vi "GetFrameRate.vi"(8 "error in (no error)":errorcluster, 11 "ICamera in":refnum<class "ICamera.lvclass">) -> (0 "error out":errorcluster, 2 "Frame Rate":u8 format="%.0x", 3 "ICamera out":refnum<class "ICamera.lvclass">)   [LabVIEW 2020, in "ICamera.lvlib" / "ICamera.lvclass"]
uses:
  ICamera.lvclass
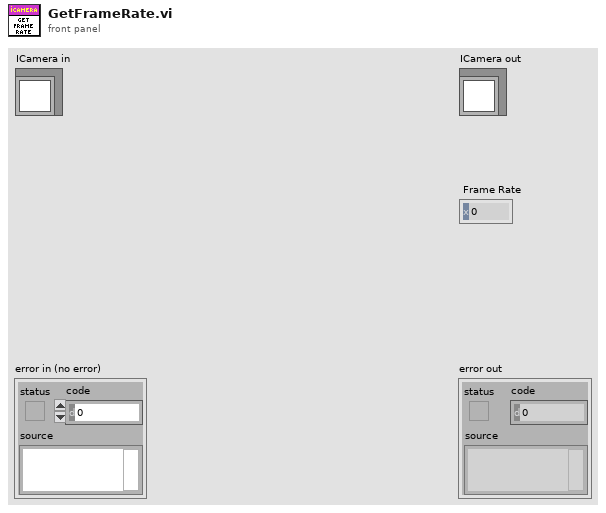
[diagram p1: front panel]
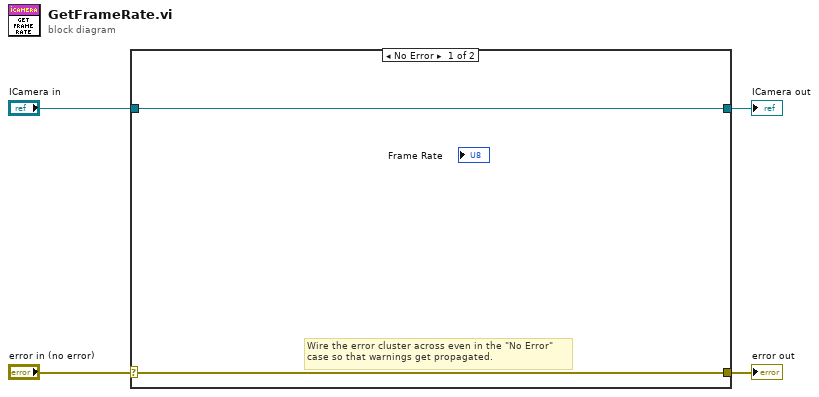
[diagram p0: block diagram]
diagram:
  n1 = case shown="No Error" "error in (no error)" {
    selector: "error in (no error)" -> [w5 w8]
    tunnel: [w5 w8] -> w3
    tunnel: [w6 w7] -> w1
    tunnel: "ICamera in" -> [w6 w7]
    frame No Error {
      # "Wire the error cluster across even in the \"No Error\"\ncase so that warnings get propagated."
    }
    frame Error {
    }
  }
  "error out" <- w3
  "ICamera out" <- w1
